vi "GeneratePause.vi"(8 "Error in":errorcluster, 11 "PauseDuration (pws)":i32) -> (0 "Error Out":errorcluster, 3 "digital waveform":digitalwaveform(waveform))   [LabVIEW 2015]
uses:
  <vilib>/Waveform/DWDTOps.llb/DWDT Boolean Array to Digital.vi
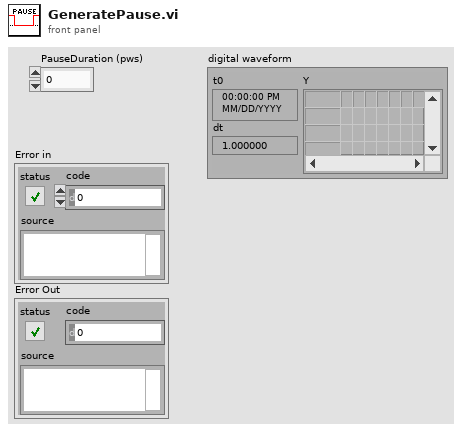
[diagram p1: front panel]
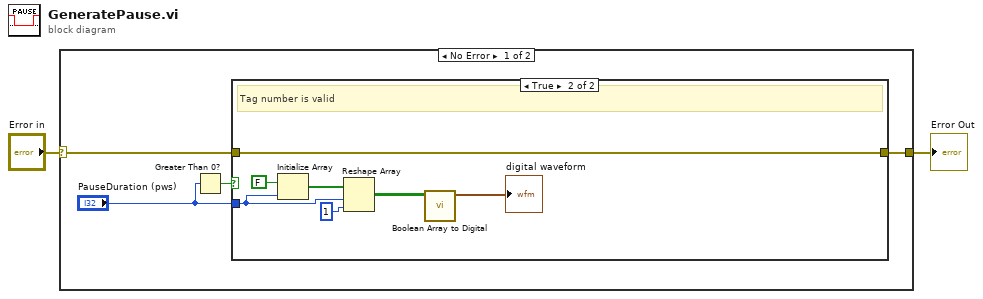
[diagram p0: block diagram]
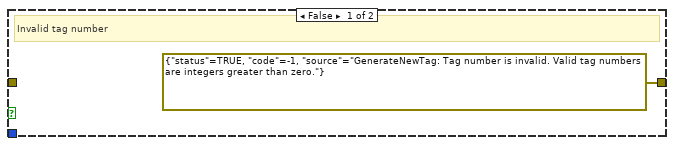
[diagram p2: hidden frame]
diagram:
  n1 = case shown="No Error" "Error in" {
    selector: "Error in" -> [w5 w15]
    tunnel: [w6 w15] -> w1
    frame No Error {
      n2 = Greater Than 0?(x="PauseDuration (pws)") -> (x > 0?=w4:bool)
      n3 = case shown="True" w4 {
        tunnel: [errorcluster {"status"=TRUE, "code"=-1, "source"="GenerateNewTag: Tag number is invalid. Valid tag numbers are integers greater than zero."} ("error IO") w13] -> w6
        tunnel: w5 -> [_ w13]
        tunnel: "PauseDuration (pws)" -> [_ w8]
        frame False {
          # "Invalid tag number"
        }
        frame True {
          # "Tag number is valid"
          n4 = Initialize Array(FALSE ("Marker on"), w8) -> (w9:bool[])
          n5 = Reshape Array(w9, w8, 1 ("dimension size")) -> (w12:bool[][])
          n6 = call-poly <vilib>:"Boolean Array to Digital.vi"("boolean array"=w12) -> ("digital waveform"=→"digital waveform":digitalwaveform)  [unwired: 9 in, 1 out]
        }
      }
    }
    frame Error {
    }
  }
  "Error Out" <- w1
